vi "Find Direction From Lidar.vi"(8 "error in (no error)":errorcluster, 11 "VISA resource name":refnum<visa-resource-name>) -> (0 "Go Straight":bool, 1 "Turn Left":bool, 2 "Turn Right":bool, 3 "VISA resource name out":refnum<visa-resource-name>, 4 "error out":errorcluster, 5 "Stop Robot":bool)   [LabVIEW 2011]
uses:
  <vilib>/robotics/Obstacle Avoidance/Simple Vector Field Histogram/Panic Range.ctl
  <vilib>/robotics/Obstacle Avoidance/Simple Vector Field Histogram/NI_Robotics_Simple Vector Field Histogram.lvlib
  <instrlib>/Hokuyo URG Series/Hokuyo URG Series.lvlib
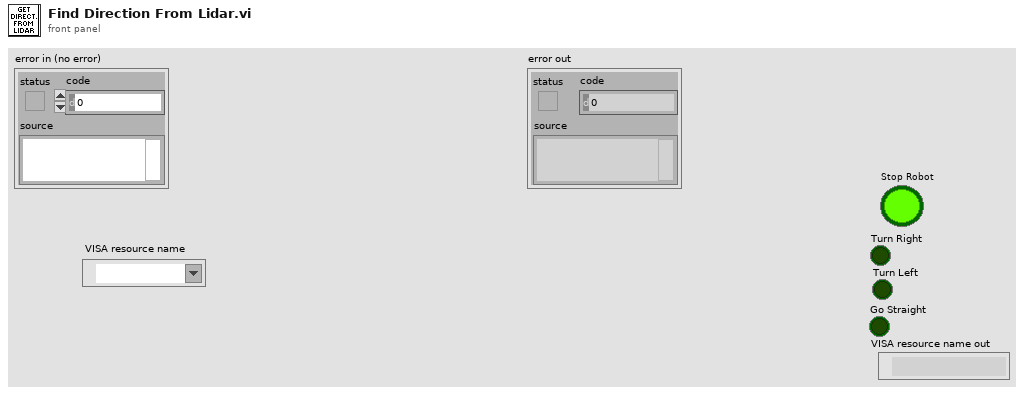
[diagram p1: front panel]
types:
  T1 = typedef "NI_Robotics_Simple Vector Field Histogram.lvlib/Panic Range.ctl" = cluster{"panic threshold distance (0)":dbl, "panic threshold angle (0)":dbl}
  T2 = typedef "NI_Robotics_Simple Vector Field Histogram.lvlib/Gap Description.ctl" = cluster{"angle to gap":dbl, "size of gap":dbl}
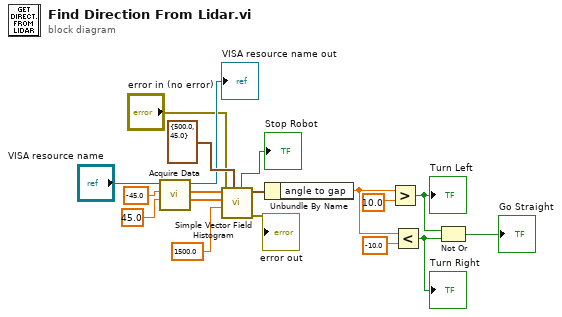
[diagram p0: block diagram]
diagram:
  n1 = call <instrlib>:"Acquire Data.vi"("End Point (120°)"=45.0, "Start Point (-120°)"=-45.0, "VISA resource name"="VISA resource name") -> ("Direction"=w17:dbl[], "Magnitude"=w18:dbl[], "VISA resource name out"=→"VISA resource name out":refnum<visa-resource-name>)  [unwired: 5 in, 1 out]
  n2 = call <vilib>:"Simple Vector Field Histogram.vi"("panic range"=T1 {"panic threshold distance (0)"=500.0, "panic threshold angle (0)"=45.0}, "error in (no error)"="error in (no error)", "distance threshold"=1500.0, "direction angles"=w17, "distances"=w18) -> ("error out"=→"error out":errorcluster, "largest gap"=w14:T2, "obstacle within panic range"=→"Stop Robot":bool)  [unwired: 2 in, 2 out]
  n3 = Unbundle By Name(w14) -> ("angle to gap"=w7:dbl)
  n4 = Greater?(x=w7, y=10.0) -> (0:w9:bool)
  "Turn Left" <- w9
  n5 = Less?(x=w7, y=-10.0) -> (x < y?=w8:bool)
  "Turn Right" <- w8
  n6 = Not Or(1:w8, 2:w9) -> (0:→"Go Straight":bool)
